vi "pigeon_ver4_1.vi"() -> ()   [LabVIEW 2017]
uses:
  <vilib>/eio/EIONode/EIONode.xnode
  <vilib>/Platform/TimedLoop/XDataNode/XDataNode.xnode
  <vilib>/Platform/TimedLoop/XDataNode/nitl_modes.ctl
  <vilib>/Platform/TimedLoop/XDataNode/XDNodeRunTimeDep.lvlib
  <vilib>/Platform/TimedLoop/XDataNode/wakeup.ctl
  <vilib>/Platform/TimedLoop/XDataNode/timing_clust.ctl
  <vilib>/rvi/DataTransferAndStorage/Container/XNode/niFpgaContainer.xnode
  <vilib>/rvi/eio/common/nirviEmuTemplateMethod_errors.vi
  <vilib>/rvi/Memory/Memory_Emulation/nirvimemoryFastEmulation.vi
  <vilib>/rvi/Memory/Memory_Emulation/nirvimemoryEmulation.vi
  <vilib>/rvi/interface/RandomDataEmulation/nirviRandomDataFpgaReadWriteTemplate.vi
  <vilib>/rvi/Analysis/common/FxpNativeNode/niFpgaFxpNative.xnode
panel:
  out "Numeric":i16
  in  "analog ramp on":bool
  out "AI2":i16
  in  "Tab Control":enum32{"pigeon"}(tab)
  in  "Emergency Stop":bool
  in  "AO0_pigeon":i16
  in  "AO7":i16
  in  "AO6":i16
  out "trigger AI1":bool
  in  "Tab Control 2":T1(tab)
  in  "square wave  on?":bool
  in  "square wave period":i32
  in  "IGBTswitch":bool caption="IGBT Switch circular"
  in  "Manual Override":bool
  in  "circular coil current":i16(slide) scale=0.0..32768.0
  in  "analog ramp period":i16
  in  "AO4":bool
  in  "analog wave shape":i16(ring) items=["Triangle", "Sawtooth", "Sin", ""]
  in  "analog ramp on  2":bool
  in  "End Current":fxp<+,16,16>
  in  "step size":i16=3
  out "ramp loop end?":bool=TRUE
  out "end val 16 bit":i16
  out "ramp start val":fxp<+,15,15>
  out "start val 16 bit":i16
  out "ctr":i16
  out "loop output val":i16
  out "FIFO size":i16
  in  "AO0":i16
  in  "AO1":i16
  in  "AO2":i16
  in  "Run program":bool
  in  "halt processor":bool
  out "control flags":i8 format="%b"
  in  "host operation":i16
  in  "address":u16
  in  "data1":u16
  in  "data2":i32
  in  "repeat program":i32
  out "IP address":i16
  out "PMT1":i16=-4740
  out "ReA":i32
  out "RegB":i16
  out "RegC":i16
  out "exttrigger":bool=TRUE
  out "AI1":i16=161
  out "RegD":i16
  in  "AO4":i16
  in  "AO3":i16
  out "Connector0/AI0":i16
  in  "AO5":i16
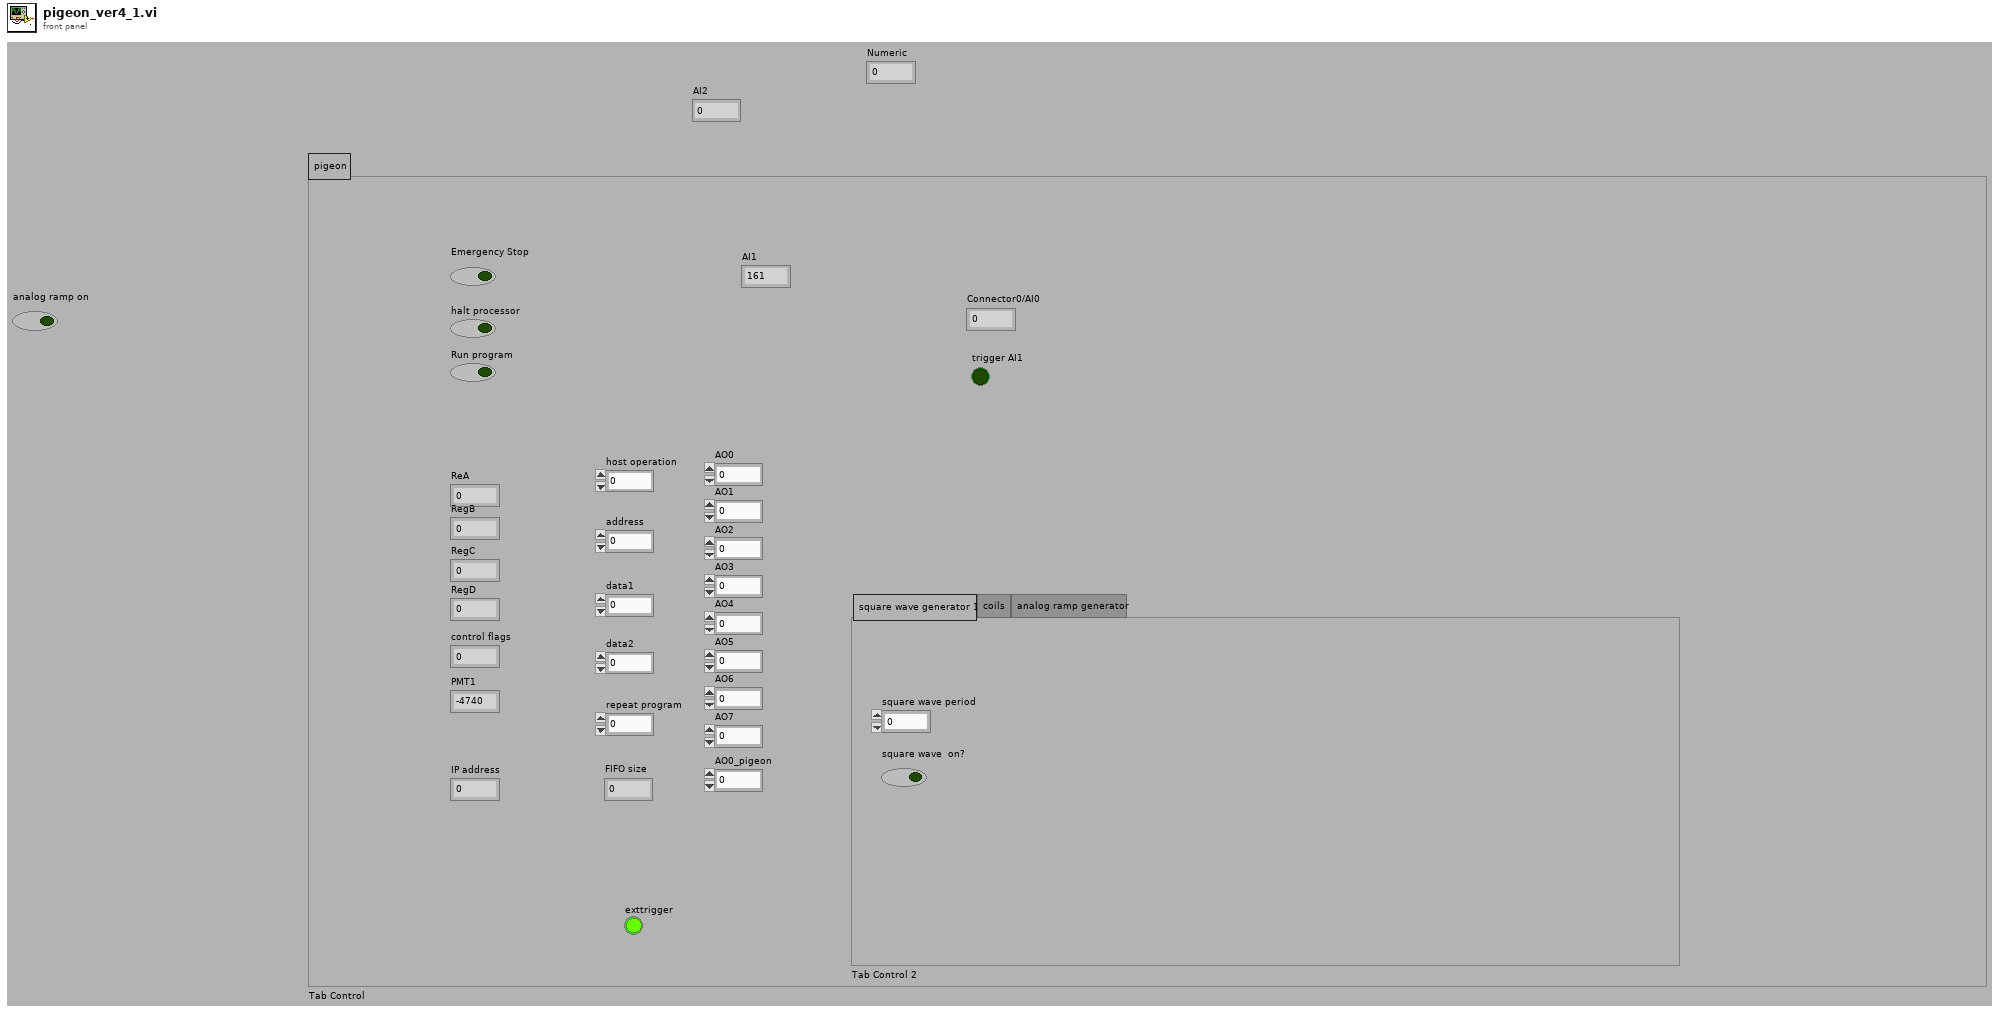
[diagram p1: front panel]
types:
  T1 = enum32{"square wave generator 1", "coils", "analog ramp generator"}
  T2 = typedef "XDNodeRunTimeDep.lvlib/timing_clust.ctl" = cluster{"Expected End [f-1]":u64, "Actual End [f-1]":u64, "Finished Late? [f-1]":bool, "Expected End [i-1]":u64, "Actual End [i-1]":u64, "Finished Late? [i-1]":bool, "Expected Start [i]":u64, "Actual Start [i]":u64, "Expected Start [f]":u64, "Actual Start [f]":u64, "Source Name":string, "Structure Name":string, "Period":i64, "Deadline":i64, "Offset":i64, "Start":i64, "Priority":i32, "Timeout":i32, "Mode":T3, "Wakeup Reason":T4, "Error":errorcluster, "Source Type":string, "Secondary Source Type":string, "Global End Time":u64, "Global Start Time":u64, "Frame Duration":u64, "Iteration Duration":u64, "Assigned CPU":i32, "I/O Scan Engine Mode":u32}
  T3 = typedef "XDNodeRunTimeDep.lvlib/nitl_modes.ctl" = enum32{"No Change", "Process missed periods, maintain original phase", "Discard missed periods, maintain original phase", "Process missed periods, ignore original phase", "Discard missed periods, ignore original phase"}
  T4 = typedef "XDNodeRunTimeDep.lvlib/wakeup.ctl" = enum32{"Normal", "Aborted", "Asynchronous wakeup", "Timing source error", "Timed loop error", "Timeout"}
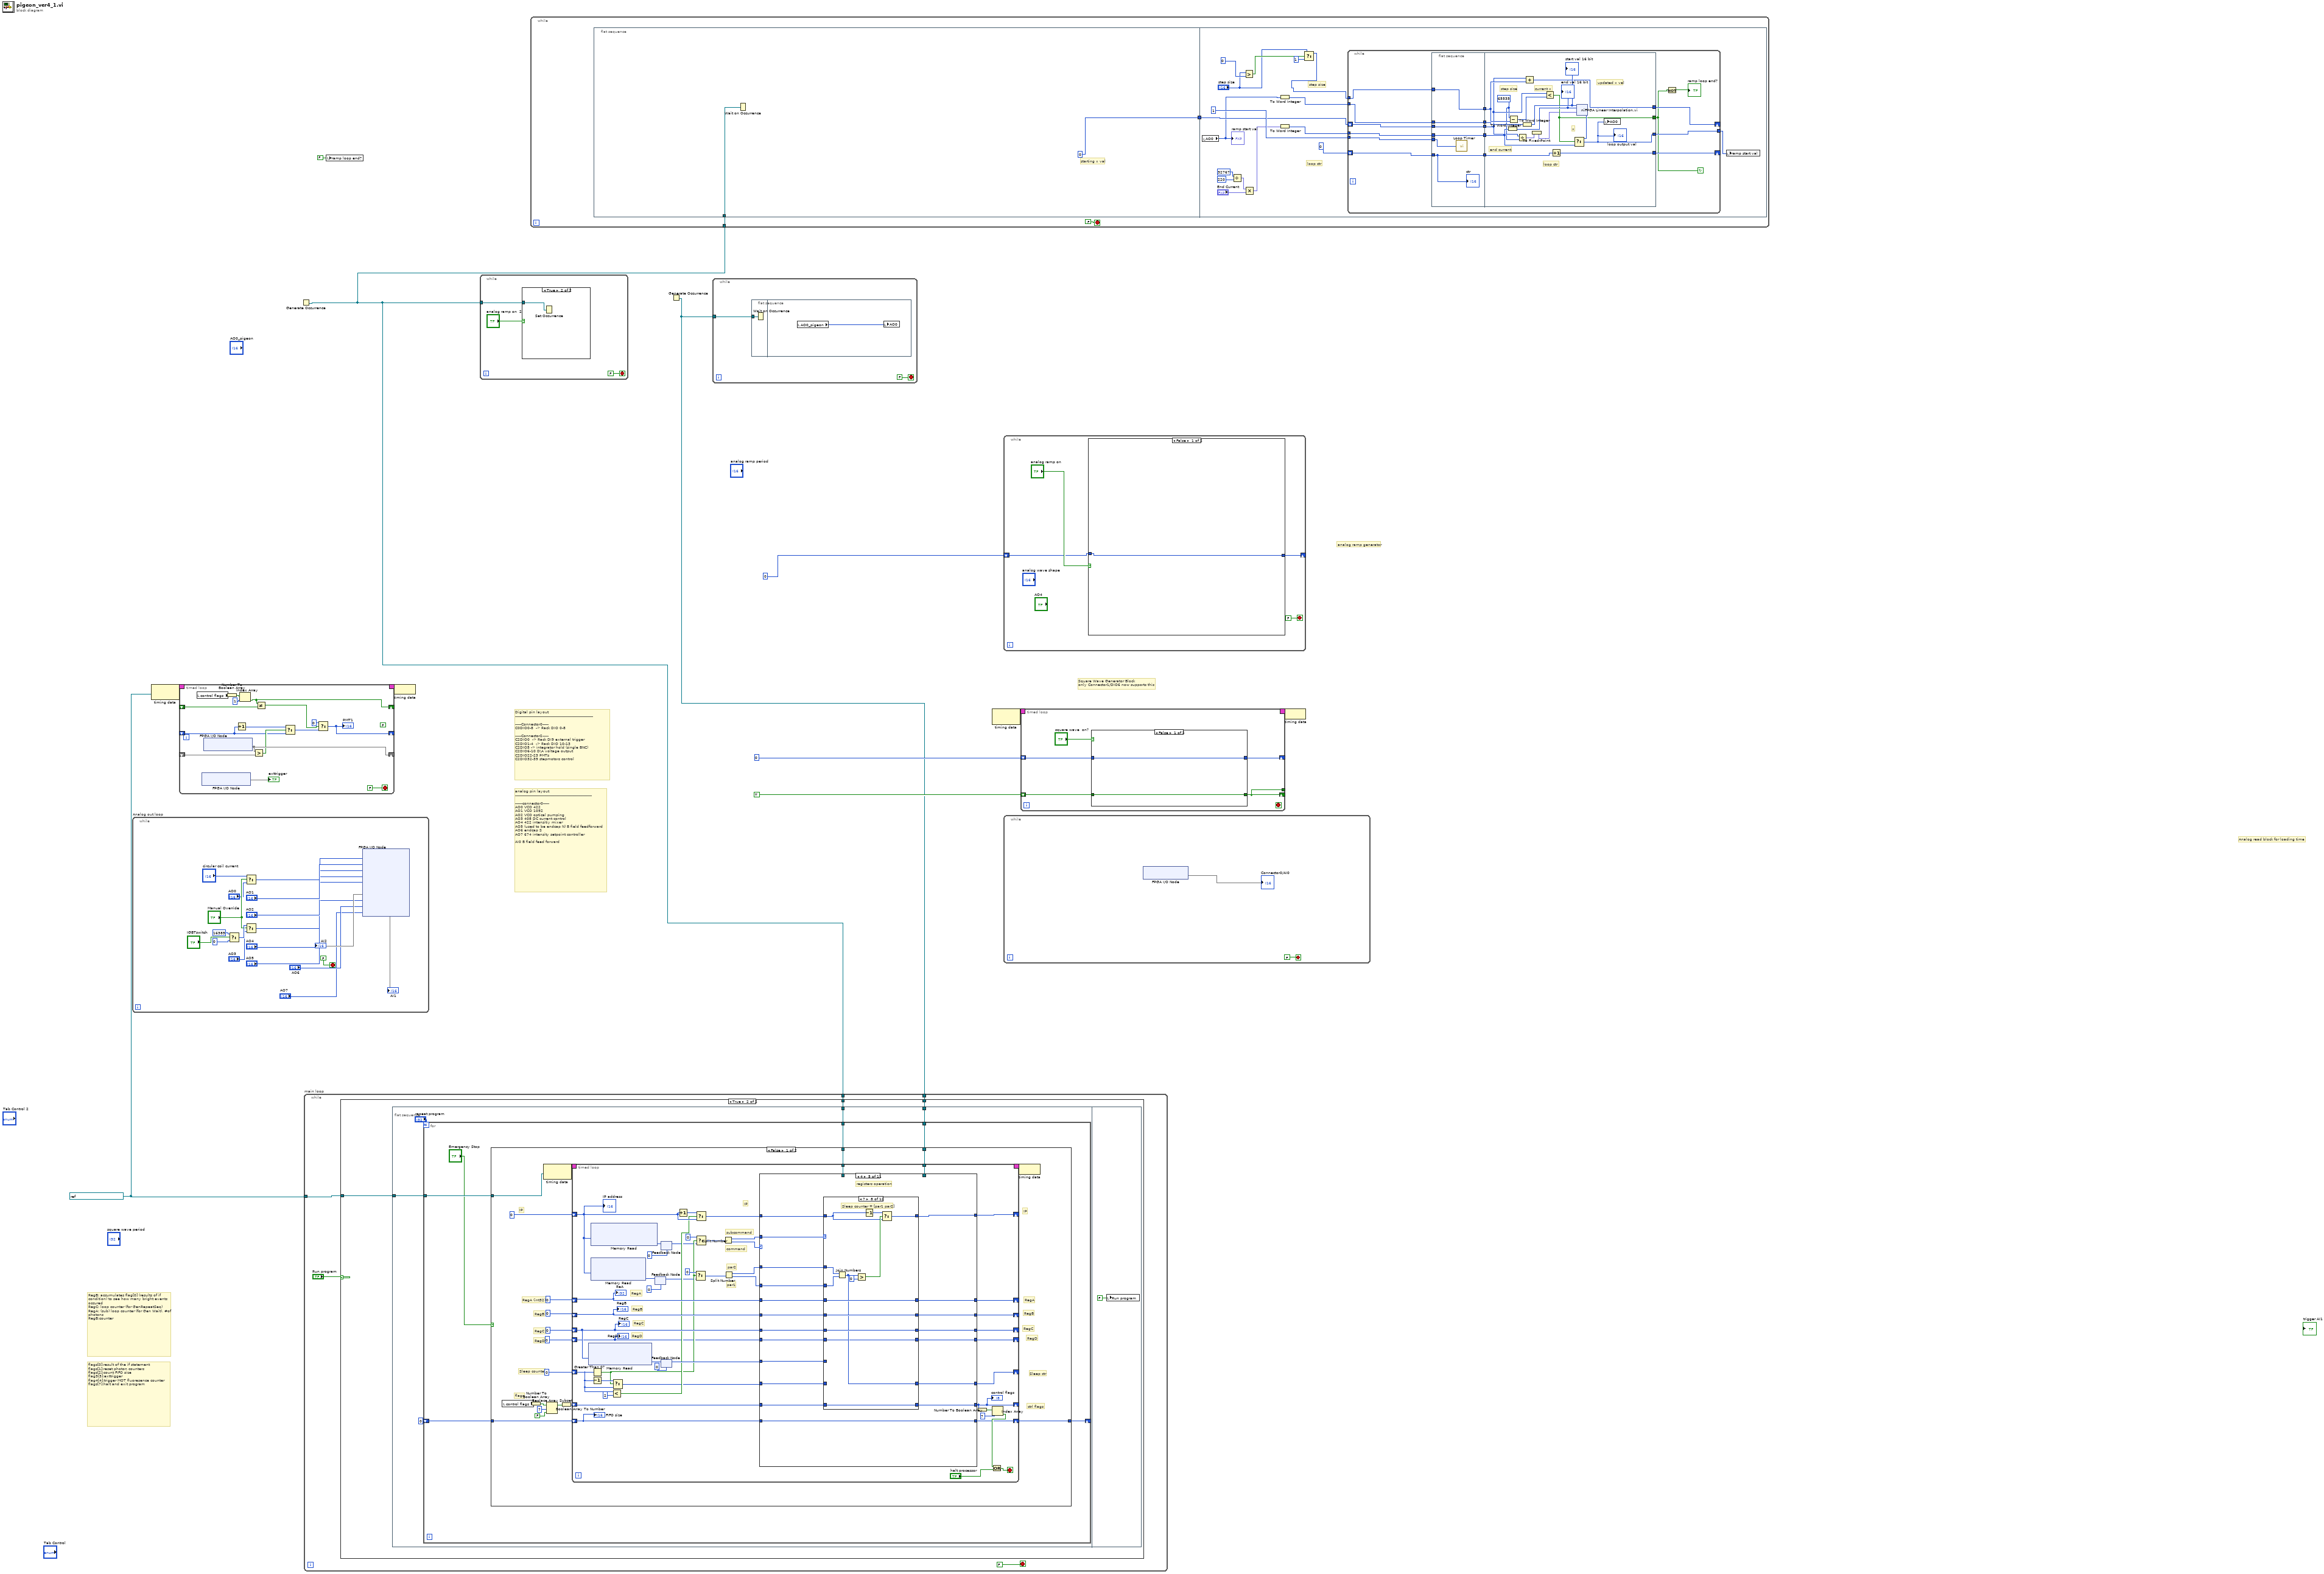
[diagram p0: block diagram]
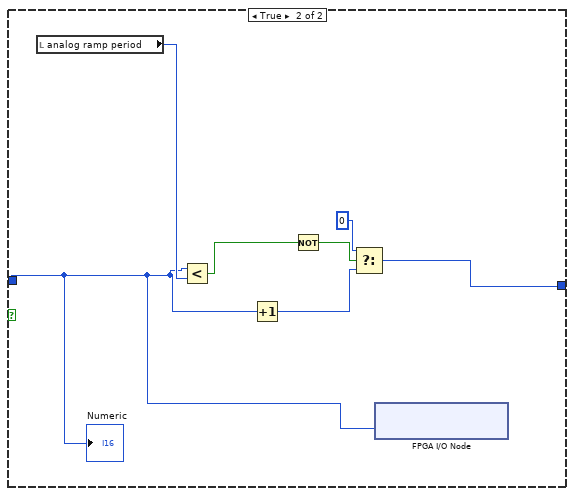
[diagram p3: hidden frame]
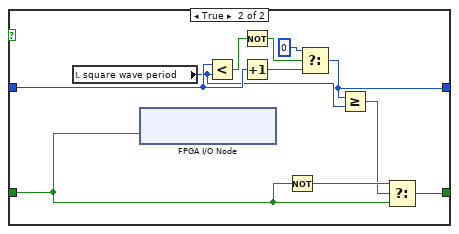
[diagram p4: hidden frame]
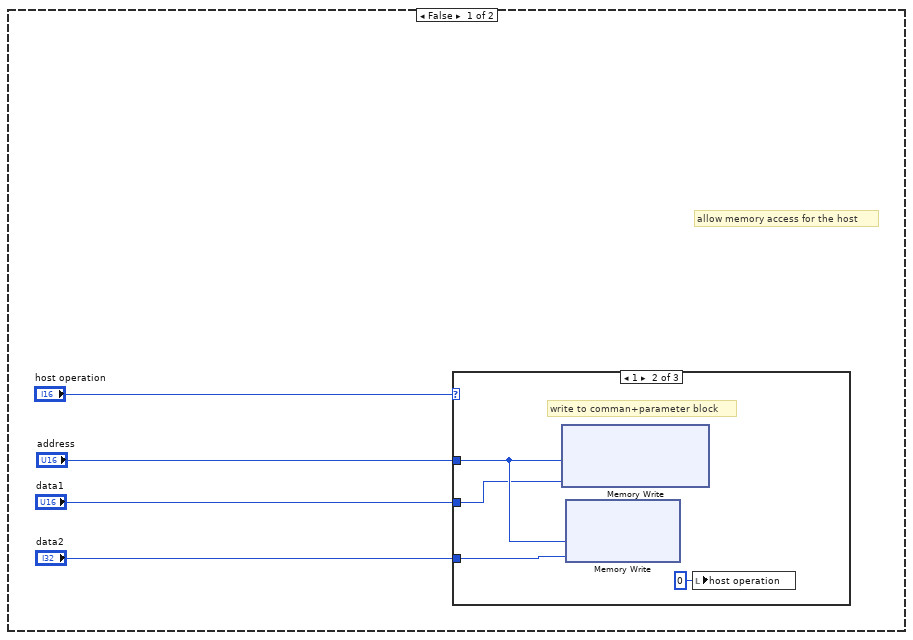
[diagram p5: hidden frame]
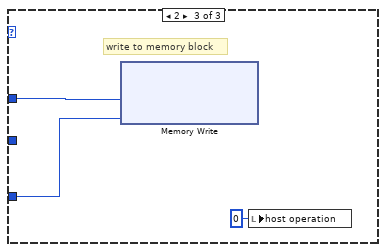
[diagram p7: hidden frame]
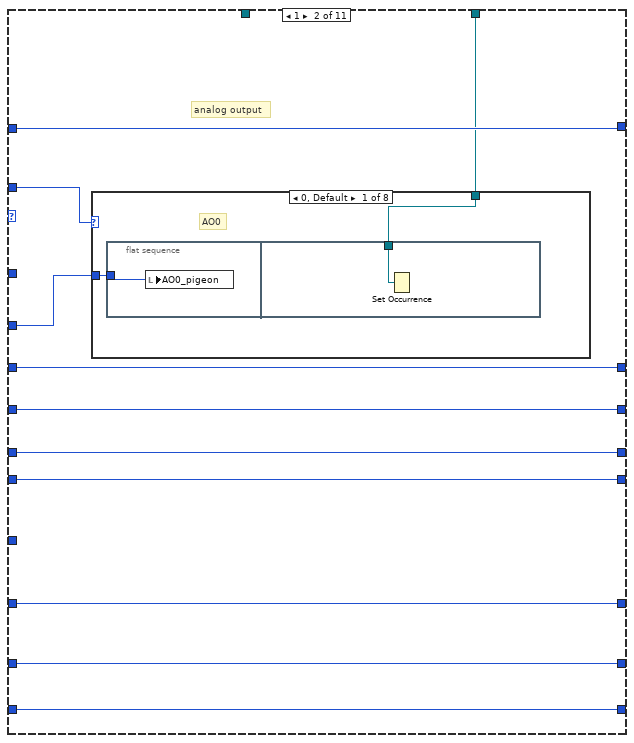
[diagram p9: hidden frame]
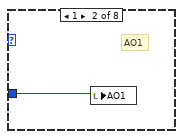
[diagram p10: hidden frame]
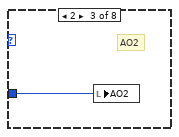
[diagram p11: hidden frame]
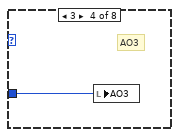
[diagram p12: hidden frame]
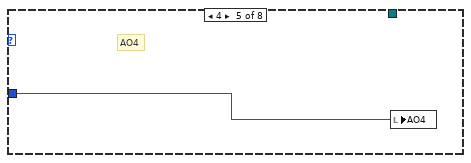
[diagram p13: hidden frame]
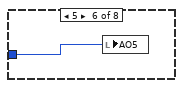
[diagram p14: hidden frame]
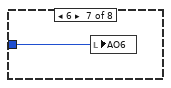
[diagram p15: hidden frame]
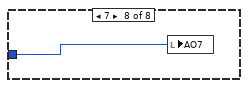
[diagram p16: hidden frame]
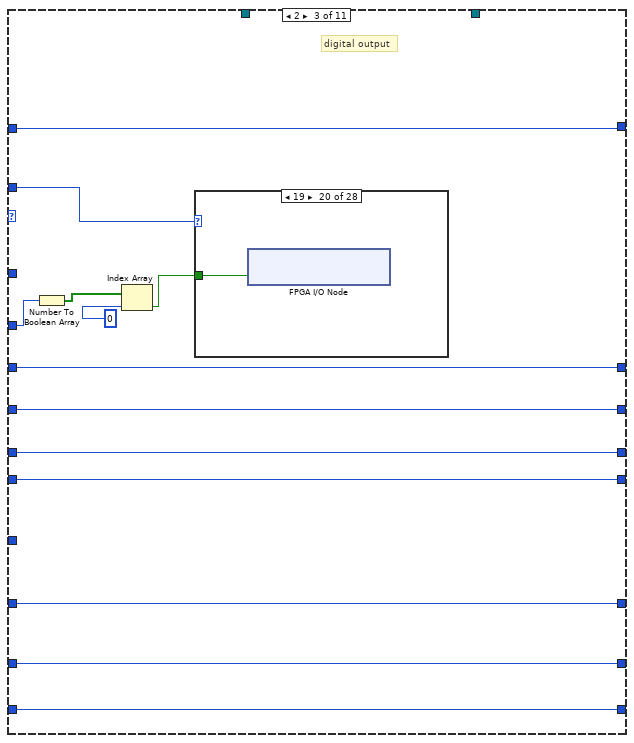
[diagram p17: hidden frame]
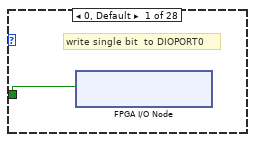
[diagram p18: hidden frame]
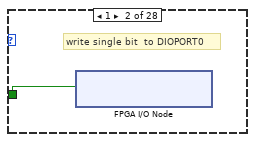
[diagram p19: hidden frame]
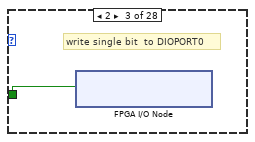
[diagram p20: hidden frame]
diagram:
  w9 = refnum<k21> "40 MHz Onboard Clock" ("FPGA Clock")
  # "analog ramp generator"
  # "Analog read block for loading time"
  # "Square Wave Generator Block\nonly Connector1/DIO6 now supports this"
  # "RegB: accumulates flag[0] (results of if condition) to see how many bright events occured\nRegC: loop counter (for GenRepeatSeq)\nRegA: (sub) loop counter (for Gen Wait), #of     photons \nRegB:counter"
  # "flags[0]:result of the if statement\nflags[1]:reset photon counters\nflags[2]:count FIFO size\nflag3[3]:exttrigger\nflag4[4]:trigger MOT fluoresence counter\nflags[7]:halt and exit program"
  # "Digital pin layout\n----------------------------------------------------------------\n\n-----Connector0-----\nC0DIO0-8  -> Rack DIO 0-8\n\n-----Connector2-----\nC2DIO0  -> Rack DI9 external trigger \nC2DIO1-4  -> Rack DIO 10-13\nC2DIO5 -> integrator hold (single BNC)\nC2DIO6-10 D\\A voltage output\nC2DIO22-23 PMTs\nC2DIO32-39 stepmotors control"
  # "analog pin layout\n---------------------------------------------------------------\n\n------connector0-----\nAO0 VCO 422\nAO1 VCO 1092\nAO2 VCO optical pumping\nAO3 408 DC current control\nAO4 422 intensitiy mixer\nAO5 (used to be endcap N) B field feedforward\nAO6 endcap S\nAO7 674 intensity setpoint controller\n\nAI0 B field feed forward"
  n1 = while "Analog out loop" {
    stop <- FALSE stop-if-true
    n2 = Select(t=i16 16385, s="IGBTswitch", f=i16 0) -> (s? t:f=w20:i16)
    n3 = Select(t="circular coil current", s="Manual Override", f="AO0") -> (s? t:f=w14:i16)
    n4 = Select(t=w20, s="Manual Override", f="AO3") -> (s? t:f=w19:i16)
    n5 = xnode "FPGA I/O Node"("Connector0/AO0"=w14, "Connector0/AO1"="AO1", "Connector0/AO2"="AO2", "Connector0/AO3"=w19, "Connector0/AO4"="AO4", "Connector0/AO5"="AO5", "Connector0/AO6"="AO6", "Connector0/AO7"="AO7") -> ("Connector0/AI1"=→"AI1", "Connector0/AI2"=→"AI2")  [unwired: 10 in, 10 out]
  }
  n6 = node-c288(w9) -> (w11:T2)
  n7 = timed-loop {
    timing: w11 -> [_]
    timing-out: [_] -> w10
    shift-right: [w44] -> _
    shift-left: _ -> [w33]
    shift-right: [w37] -> _
    shift-left: _ -> [w46]
    shift-right: [w39] -> _
    shift-left: _ -> [w40]
    stop <- FALSE stop-if-true
    (unwired) FALSE
    n8 = local read "control flags"() -> (w41:i8)
    n9 = xnode "FPGA I/O Node"() -> ("Connector2/DIO0"=→"exttrigger")  [unwired: 1 in, 1 out]
    n10 = xnode "FPGA I/O Node"() -> ("Connector0/DIO0"=w37)  [unwired: 1 in, 1 out]
    n11 = Number To Boolean Array(number=w41) -> (Boolean array=w42:bool[])
    n12 = Increment(x=w33) -> (x+1=w34:u16)
    n13 = Index Array(array=w42, index=1) -> (element=w39:bool)
    n14 = Greater?(x=w37, y=w46) -> (0:w36:bool)
    n15 = Not Equal?(x=w39, y=w40) -> (x != y?=w31:bool)
    n16 = Select(t=w34, s=w36, f=w33) -> (s? t:f=w45:u16)
    n17 = Select(t=u16 0, s=w31, f=w45) -> (s? t:f=w44:u16)
    "PMT1" <- w44
  }
  n18 = Generate Occurrence() -> (w2:refnum<k4>)
  n19 = local write "ramp loop end?"(FALSE ("ramp loop end?")) -> ()
  n20 = node-c288(w10) -> ()
  n21 = while {
    tunnel: w2 -> [w50]
    stop <- FALSE stop-if-true
    n22 = case shown="True" "analog ramp on  2" {
      tunnel: w50 -> [_ w52]
      frame False {
      }
      frame True {
        n23 = Set Occurrence(w52) -> ()
      }
    }
  }
  n24 = while {
    tunnel: w2 -> [w53]
    stop <- FALSE stop-if-true
    n25 = flat-sequence {
      tunnel: [u16 0] -> w54
      tunnel: w53 -> [w56]
      tunnel: w54 -> [w67]
      frame #0 {
        # "starting x val"
        n26 = Wait on Occurrence(2:w56) -> ()  [unwired: 2 in, 1 out]
      }
      frame #1 {
        # "loop ctr"
        # "step size"
        n27 = local read "AO0"() -> (w58:i16)
        "ramp start val" <- w58
        n28 = Divide(x=i16 32767, y=i16 220) -> (x/y=w72:fxp<+,16,16>)
        n29 = Greater?(x="step size", y=i16 0) -> (0:w62:bool)
        n30 = Multiply(x=w72, y="End Current") -> (x*y=w65:fxp<+,32,32>)
        n31 = To Word Integer(number=w58) -> (16bit integer=w70:i16)
        n32 = To Word Integer(number=w65) -> (16bit integer=w69:i16)
        n33 = Select(t="step size", s=w62, f=i16 1) -> (s? t:f=w59:i16)
        n34 = while {
          tunnel: w59 -> [w78]
          tunnel: w70 -> [w90]
          tunnel: w69 -> [w89]
          shift-right: [w88] -> _
          shift-left: w67 -> [w77]
          tunnel: u32 1 ("Update Period (uSec)") -> [w87]
          shift-right: [w81] -> _
          shift-left: i16 0 -> [w79]
          tunnel: [w80] -> w66
          stop <- w76 continue-if-true
          n35 = flat-sequence {
            tunnel: w78 -> [w95]
            tunnel: [w95] -> w86
            tunnel: w90 -> [w94]
            tunnel: [w94] -> w85
            tunnel: w89 -> [w93]
            tunnel: [w93] -> w84
            tunnel: w77 -> [w92]
            tunnel: [w92] -> w83
            tunnel: w87 -> [w96]
            tunnel: w79 -> [w91]
            tunnel: [w91] -> w82
            tunnel: w86 -> [w104]
            tunnel: w85 -> [w112]
            tunnel: w84 -> [w102]
            tunnel: w83 -> [w100]
            tunnel: [w105] -> w76
            tunnel: [w106] -> w88
            tunnel: [w108] -> w81
            tunnel: w82 -> [w107]
            tunnel: [w97] -> w80
            frame #0 {
              n36 = call "Loop Timer"("Count(uSec)"=w96) -> ()  [unwired: 1 out]
              "ctr" <- w91
            }
            frame #1 {
              w98 = u16 65535 ("x")
              # "current x"
              # "end current"
              # "x"
              # "loop ctr"
              # "updated x val"
              # "step size"
              n37 = To Word Integer(number=w102) -> (16bit integer=w109:i16)
              "end val 16 bit" <- w109
              n38 = Subtract(x=w98, y=w104) -> (x-y=w103:u16)
              n39 = Divide(x=w100, y=w98) -> (x/y=w99:fxp<+,16,0>)
              n40 = To Word Integer(number=w112) -> (16bit integer=w110:i16)
              "start val 16 bit" <- w110
              n41 = Add(x=w100, y=w104) -> (x+y=w106:u16)
              n42 = To Fixed-Point(number=w99) -> (fixed-point=w101:fxp<+,16,0>)  [unwired: 1 in]
              n43 = Less?(x=w100, y=w103) -> (x < y?=w105:bool)
              n44 = Increment(x=w107) -> (x+1=w108:i16)
              n45 = xnode ("niFPGA Linear Interpolation.vi")("y0"=w110, "y1"=w109, "x"=w101) -> ("y"=w111:i16)
              n46 = Select(t=w111, s=w105, f=w102) -> (s? t:f=w97:i16)
              "loop output val" <- w97
              n47 = local write "AO0"(w97) -> ()
            }
          }
          n48 = Not(x=w76) -> (.not. x?=→"ramp loop end?":bool)
        }
        n49 = local write "ramp start val"(w66) -> ()
      }
    }
  }
  n50 = Generate Occurrence() -> (w1:refnum<k4>)
  n51 = while "main loop" {
    tunnel: w9 -> [w126]
    tunnel: w2 -> [w125]
    tunnel: w1 -> [w124]
    stop <- FALSE ("stop") stop-if-true
    n52 = case shown="True" "Run program" {
      tunnel: w126 -> [_ w142]
      tunnel: w125 -> [_ w141]
      tunnel: w124 -> [_ w140]
      frame False {
        # "allow memory access for the host"
        n53 = case shown="1" "host operation" {
          tunnel: "address" -> [_ w134 w139]
          tunnel: "data1" -> [_ w133 _]
          tunnel: "data2" -> [_ w136 w137]
          frame 0, Default {
          }
          frame 1 {
            # "write to comman+parameter block"
            n54 = xnode ("Memory Write")("Address"=w134, "Data"=w133) -> ()  [unwired: 1 in, 1 out]
            n55 = xnode ("Memory Write")("Address"=w134, "Data"=w136) -> ()  [unwired: 1 in, 1 out]
            n56 = local write "host operation"(i16 0 ("host operation")) -> ()
          }
          frame 2 {
            # "write to memory block"
            n57 = xnode ("Memory Write")("Address"=w139, "Data"=w137) -> ()  [unwired: 1 in, 1 out]
            n58 = local write "host operation"(i16 0 ("host operation")) -> ()
          }
        }
      }
      frame True {
        n59 = flat-sequence {
          tunnel: w142 -> [w146]
          tunnel: w141 -> [w144]
          tunnel: w140 -> [w143]
          frame #0 {
            n60 = for {
              N: "repeat program" -> [_]
              tunnel: w146 -> [w153]
              shift-right: [w151] -> _
              shift-left: i16 0 -> [w152]
              tunnel: w144 -> [w150]
              tunnel: w143 -> [w149]
              n61 = case shown="False" "Emergency Stop" {
                tunnel: w153 -> [w166 _]
                tunnel: w152 -> [w158 w630]
                tunnel: [w157 w630] -> w151
                tunnel: w150 -> [w155 _]
                tunnel: w149 -> [w154 _]
                frame False {
                  # "ctrl flags"
                  # "Sleep ctr"
                  # "RegD"
                  # "RegD"
                  # "Sleep counter"
                  # "flags"
                  # "RegC"
                  # "RegB"
                  # "RegA"
                  # "RegC"
                  # "RegB"
                  # "RegA (int32)"
                  # "IP"
                  # "IP"
                  n62 = local read "control flags"() -> (w161:i8)
                  n63 = Number To Boolean Array(number=w161) -> (Boolean array=w165:bool[])
                  n64 = node-c288(w166) -> (w172:T2)
                  n65 = Replace Array Subset(array=w165, new element=FALSE ("new element/subarray"), index=7) -> (w163:bool[])
                  n66 = Boolean Array To Number(Boolean array=w163) -> (number=w164:u8)
                  n67 = timed-loop {
                    timing: w172 -> [_]
                    timing-out: [_] -> w171
                    shift-right: [w209] -> _
                    shift-left: i16 0 -> [w192]
                    shift-right: [w205] -> _
                    shift-left: 0 -> [w201]
                    shift-right: [w217] -> _
                    shift-left: i16 0 -> [w208]
                    shift-right: [w216] -> _
                    shift-left: i16 0 -> [w200]
                    shift-right: [w206] -> _
                    shift-left: w164 -> [w207]
                    shift-right: [w199] -> _
                    shift-left: i16 0 -> [w190]
                    shift-right: [w181] -> w157
                    shift-left: w158 -> [w180]
                    shift-right: [w178] -> _
                    shift-left: i16 0 -> [w179]
                    tunnel: w155 -> [w174]
                    tunnel: w154 -> [w173]
                    stop <- w212 stop-if-true
                    # "RegD"
                    # "IP"
                    # "RegC"
                    # "RegB"
                    # "RegA"
                    # "par1"
                    # "par2"
                    # "subcommand"
                    # "command"
                    n68 = xnode ("Memory Read")("Address"=w200) -> ("Data"=w204:i16)  [unwired: 2 in, 2 out]
                    n69 = xnode ("Memory Read")("Address"=w192) -> ("Data"=w187:u16)  [unwired: 1 in, 1 out]
                    n70 = xnode ("Memory Read")("Address"=w192) -> ("Data"=w183:i32)  [unwired: 1 in, 1 out]
                    n71 = Greater Than 0?(x=w190) -> (x > 0?=w185:bool)
                    n72 = Decrement(x=w190) -> (x-1=w191:u32)
                    n73 = Less?(x=w190, y=u32 2) -> (x < y?=w189:bool)
                    n74 = Select(t=w191, s=w185, f=w190) -> (s? t:f=w188:u32)
                    n75 = feedback-in #1(w183) -> ()
                    n76 = feedback #1(u32 0 ("Data")) -> (w182:u32)
                    n77 = feedback-in #2(w204) -> ()
                    n78 = feedback #2(0) -> (w203:i32)
                    n79 = feedback-in #3(w187) -> ()
                    n80 = feedback #3(u16 0 ("Data")) -> (w184:u16)
                    n81 = Increment(x=w192) -> (x+1=w193:u16)
                    n82 = Select(t=0, s=w185, f=w182) -> (s? t:f=w196:u32)
                    n83 = Select(t=w193, s=w189, f=w192) -> (s? t:f=w198:u16)
                    n84 = Select(t=u16 0, s=w185, f=w184) -> (s? t:f=w197:u16)
                    n85 = Split Number(x=w197) -> (hi(x)=w218:u8, lo(x)=w219:u8)
                    n86 = Split Number(x=w196) -> (hi(x)=w210:u16, lo(x)=w211:u16)
                    n87 = case shown="4" w219 {
                      tunnel: w211 -> [_ w237 w254 _ w334 w454 w528 _ _ w588 _]
                      tunnel: w210 -> [_ _ _ _ w327 w453 w527 _ _ w589 _]
                      tunnel: w218 -> [_ w238 w262 w301 w335 w458 _ w546 _ w570 _]
                      tunnel: w201 -> [w227 w236 w261 w293 w333 w455 w532 w550 w566 w587 w617]
                      tunnel: [w227 w236 w261 w293 w330 w455 w532 w550 w566 w586 w617] -> w205
                      tunnel: w208 -> [w226 w235 w260 w292 w332 w456 w533 w549 w569 w585 w618]
                      tunnel: w200 -> [w225 w234 w259 w299 w331 w457 w534 w548 w568 w583 w619]
                      tunnel: [w226 w235 w260 w291 w329 w456 w533 w549 w569 w584 w618] -> w217
                      tunnel: [w225 w234 w259 w299 w328 w457 w534 w548 w568 w582 w619] -> w216
                      tunnel: [w223 w233 w258 w300 w323 w461 w526 w552 w567 w572 w616] -> w209
                      tunnel: w198 -> [w223 w233 w258 w300 w324 w461 _ w552 w567 w573 w616]
                      tunnel: [w224 w232 w257 w297 w325 w460 w525 w541 w563 w576 w622] -> w206
                      tunnel: w207 -> [w224 w232 w257 w298 w326 w459 w525 w540 w562 w577 w622]
                      tunnel: w203 -> [_ _ _ _ w317 w452 _ _ _ _ _]
                      tunnel: w188 -> [w222 w231 w252 w296 w322 w451 w524 w538 w559 w579 w623]
                      tunnel: [w222 w231 w252 w296 w321 w451 w524 w538 w559 w578 w623] -> w199
                      tunnel: w180 -> [w221 w230 w251 w295 w320 w450 w523 w537 w558 w574 w621]
                      tunnel: [w221 w230 w251 w295 w320 w450 w523 w536 w558 w575 w621] -> w181
                      tunnel: w179 -> [w220 w229 w250 w294 w319 w449 w522 w535 w557 w581 w620]
                      tunnel: [w220 w229 w250 w294 w318 w449 w522 w535 w557 w580 w620] -> w178
                      tunnel: w174 -> [_ _ _ _ _ _ _ _ _ w571 _]
                      tunnel: w173 -> [_ w228 _ _ _ _ _ _ _ _ _]
                      frame 0, Default {
                      }
                      frame 1 {
                        # "analog output"
                        n88 = case shown="0, Default" w238 {
                          tunnel: w237 -> [w240 w243 w244 w245 w246 w247 w248 w249]
                          tunnel: w228 -> [w239 _ _ _ _ _ _ _]
                          frame 0, Default {
                            # "AO0"
                            n89 = flat-sequence {
                              tunnel: w240 -> [w241]
                              tunnel: w239 -> [w242]
                              frame #0 {
                                n90 = local write "AO0_pigeon"(w241) -> ()
                              }
                              frame #1 {
                                n91 = Set Occurrence(w242) -> ()
                              }
                            }
                          }
                          frame 1 {
                            # "AO1"
                            n92 = local write "AO1"(w243) -> ()
                          }
                          frame 2 {
                            # "AO2"
                            n93 = local write "AO2"(w244) -> ()
                          }
                          frame 3 {
                            # "AO3"
                            n94 = local write "AO3"(w245) -> ()
                          }
                          frame 4 {
                            # "AO4"
                            n95 = local write "AO4"(w246) -> ()
                          }
                          frame 5 {
                            n96 = local write "AO5"(w247) -> ()
                          }
                          frame 6 {
                            n97 = local write "AO6"(w248) -> ()
                          }
                          frame 7 {
                            n98 = local write "AO7"(w249) -> ()
                          }
                        }
                      }
                      frame 2 {
                        # "digital output"
                        n99 = Number To Boolean Array(number=w254) -> (Boolean array=w255:bool[])
                        n100 = Index Array(array=w255, index=0) -> (element=w253:bool)
                        n101 = case shown="19" w262 {
                          tunnel: w253 -> [w263 w264 w265 w266 w267 w268 w269 w270 w271 w272 w273 w274 w275 w276 w277 w278 w279 w280 w281 w282 w283 w284 w285 w286 w287 w288 w289 w290]
                          frame 0, Default {
                            # "write single bit  to DIOPORT0"
                            n102 = xnode "FPGA I/O Node"("Connector1/DIO0"=w263) -> ()  [unwired: 1 in, 1 out]
                          }
                          frame 1 {
                            # "write single bit  to DIOPORT0"
                            n103 = xnode "FPGA I/O Node"("Connector1/DIO1"=w264) -> ()  [unwired: 1 in, 1 out]
                          }
                          frame 2 {
                            # "write single bit  to DIOPORT0"
                            n104 = xnode "FPGA I/O Node"("Connector1/DIO2"=w265) -> ()  [unwired: 1 in, 1 out]
                          }
                          frame 3 {
                            # "write single bit  to DIOPORT0"
                            n105 = xnode "FPGA I/O Node"("Connector1/DIO3"=w266) -> ()  [unwired: 1 in, 1 out]
                          }
                          frame 4 {
                            # "write single bit  to DIOPORT0"
                            n106 = xnode "FPGA I/O Node"("Connector1/DIO4"=w267) -> ()  [unwired: 1 in, 1 out]
                          }
                          frame 5 {
                            # "write single bit  to DIOPORT0"
                            n107 = xnode "FPGA I/O Node"("Connector1/DIO5"=w268) -> ()  [unwired: 1 in, 1 out]
                          }
                          frame 6 {
                            # "write single bit  to DIOPORT0"
                            n108 = xnode "FPGA I/O Node"("Connector1/DIO6"=w269) -> ()  [unwired: 1 in, 1 out]
                          }
                          frame 7 {
                            # "write single bit  to DIOPORT0"
                            n109 = xnode "FPGA I/O Node"("Connector1/DIO7"=w270) -> ()  [unwired: 1 in, 1 out]
                          }
                          frame 8 {
                            # "write single bit  to DIOPORT0"
                            n110 = xnode "FPGA I/O Node"("Connector1/DIO8"=w271) -> ()  [unwired: 1 in, 1 out]
                          }
                          frame 9 {
                            n111 = xnode "FPGA I/O Node"("Connector1/DIO9"=w272) -> ()  [unwired: 1 in, 1 out]
                          }
                          frame 10 {
                            n112 = xnode "FPGA I/O Node"("Connector1/DIO10"=w273) -> ()  [unwired: 1 in, 1 out]
                          }
                          frame 11 {
                            n113 = xnode "FPGA I/O Node"("Connector1/DIO11"=w274) -> ()  [unwired: 1 in, 1 out]
                          }
                          frame 12 {
                            n114 = xnode "FPGA I/O Node"("Connector1/DIO12"=w275) -> ()  [unwired: 1 in, 1 out]
                          }
                          frame 13 {
                            n115 = xnode "FPGA I/O Node"("Connector1/DIO13"=w276) -> ()  [unwired: 1 in, 1 out]
                          }
                          frame 14 {
                            n116 = xnode "FPGA I/O Node"("Connector1/DIO14"=w277) -> ()  [unwired: 1 in, 1 out]
                          }
                          frame 15 {
                            n117 = xnode "FPGA I/O Node"("Connector1/DIO15"=w278) -> ()  [unwired: 1 in, 1 out]
                          }
                          frame 16 {
                            n118 = xnode "FPGA I/O Node"("Connector1/DIO16"=w279) -> ()  [unwired: 1 in, 1 out]
                          }
                          frame 17 {
                            n119 = xnode "FPGA I/O Node"("Connector1/DIO17"=w280) -> ()  [unwired: 1 in, 1 out]
                          }
                          frame 18 {
                            n120 = xnode "FPGA I/O Node"("Connector1/DIO18"=w281) -> ()  [unwired: 1 in, 1 out]
                          }
                          frame 19 {
                            n121 = xnode "FPGA I/O Node"("Connector1/DIO19"=w282) -> ()  [unwired: 1 in, 1 out]
                          }
                          frame 20 {
                            n122 = xnode "FPGA I/O Node"("Connector2/DIO12"=w283) -> ()  [unwired: 1 in, 1 out]
                          }
                          frame 21 {
                            n123 = xnode "FPGA I/O Node"("Connector2/DIO17"=w284) -> ()  [unwired: 1 in, 1 out]
                          }
                          frame 22 {
                            n124 = xnode "FPGA I/O Node"("Connector2/DIO19"=w285) -> ()  [unwired: 1 in, 1 out]
                          }
                          frame 23 {
                            n125 = xnode "FPGA I/O Node"("Connector2/DIO18"=w286) -> ()  [unwired: 1 in, 1 out]
                          }
                          frame 24 {
                            n126 = xnode "FPGA I/O Node"("Connector2/DIO21"=w287) -> ()  [unwired: 1 in, 1 out]
                          }
                          frame 25 {
                            n127 = xnode "FPGA I/O Node"("Connector2/DIO24"=w288) -> ()  [unwired: 1 in, 1 out]
                          }
                          frame 26 {
                            n128 = xnode "FPGA I/O Node"("Connector2/DIO25"=w289) -> ()  [unwired: 1 in, 1 out]
                          }
                          frame 27 {
                            n129 = xnode "FPGA I/O Node"("Connector2/DIO20"=w290) -> ()  [unwired: 1 in, 1 out]
                          }
                        }
                      }
                      frame 3 {
                        # "photon counting"
                        n130 = case shown="3" w301 {
                          tunnel: [w302 w304 w316] -> w291
                          tunnel: w292 -> [w302 w305 w316]
                          tunnel: w298 -> [w303 w307 w314]
                          tunnel: [w303 w307 w313] -> w297
                          frame 2, Default {
                          }
                          frame 1 {
                            # "PMT1"
                            n131 = local read "PMT1"() -> (w306:i16)
                            n132 = Add(x=w306, y=w305) -> (x+y=w304:u16)
                          }
                          frame 3 {
                            # "Reset  photon counter"
                            # "make a Not gate of flag(1)"
                            n133 = Number To Boolean Array(number=w314) -> (Boolean array=w311:bool[])
                            n134 = Index Array(array=w311, index=1) -> (element=w309:bool)
                            n135 = Not(x=w309) -> (.not. x?=w308:bool)
                            n136 = Replace Array Subset(array=w311, new element=w308, index=1) -> (w312:bool[])
                            n137 = Boolean Array To Number(Boolean array=w312) -> (number=w313:u8)
                          }
                        }
                      }
                      frame 4 {
                        # "registers operation"
                        n138 = case shown="7" w335 {
                          tunnel: w334 -> [w341 w351 w358 _ _ _ _ w400 _ _ w427 w440]
                          tunnel: w333 -> [_ w350 w357 w364 w372 w380 w384 w405 w416 w422 w432 w445]
                          tunnel: w332 -> [w344 _ w356 w363 w374 w379 w392 w404 w415 w418 w430 w443]
                          tunnel: w331 -> [w343 w349 _ w366 w373 _ w385 w403 w414 w421 w431 w444]
                          tunnel: [w340 w350 w357 w364 w371 w380 w384 w405 w416 w422 w432 w445] -> w330
                          tunnel: [w344 w351 w356 w363 w374 w379 w391 w404 w415 w420 w430 w443] -> w329
                          tunnel: [w343 w349 w358 w365 w373 w379 w385 w403 w414 w421 w431 w444] -> w328
                          tunnel: w327 -> [w342 _ _ _ _ _ _ w401 _ _ _ w439]
                          tunnel: w326 -> [w339 w348 w355 w362 w370 w378 w386 w402 w413 w425 w435 w448]
                          tunnel: [w339 w348 w355 w362 w370 w378 w386 w402 w413 w425 w435 w448] -> w325
                          tunnel: w324 -> [w338 w347 w354 w361 w369 w377 w383 w394 w408 w424 w434 w447]
                          tunnel: [w338 w347 w354 w361 w369 w377 w383 w397 w411 w424 w434 w447] -> w323
                          tunnel: w322 -> [w337 w346 w353 w360 w368 w376 w382 _ _ w423 w433 w446]
                          tunnel: [w337 w346 w353 w360 w368 w376 w382 w398 w406 w423 w433 w446] -> w321
                          tunnel: w319 -> [w336 w345 w352 w359 w367 w375 w381 w393 w407 w417 _ w438]
                          tunnel: [w336 w345 w352 w359 w367 w375 w381 w393 w407 w417 w428 w437] -> w318
                          tunnel: w317 -> [_ _ _ _ _ _ _ _ w406 _ _ _]
                          frame 0, Default {
                            # "Set par1,2 to RegA"
                            n139 = Join Numbers(hi=w342, lo=w341) -> ((hi.lo)=w340:u32)
                          }
                          frame 1 {
                            # "Set par1 to RegB"
                          }
                          frame 2 {
                            # "Set par1 to RegC"
                          }
                          frame 3 {
                            # "increase RegC by 1"
                            n140 = Increment(x=w366) -> (x+1=w365:u16)
                          }
                          frame 4 {
                            # "increase RegA by 1"
                            n141 = Increment(x=w372) -> (x+1=w371:u32)
                          }
                          frame 5 {
                            # "Set regC to regB"
                          }
                          frame 6 {
                            # "regB<-regB+flags[0]"
                            n142 = Number To Boolean Array(number=w386) -> (Boolean array=w390:bool[])
                            n143 = Index Array(array=w390, index=0) -> (element=w388:bool)
                            n144 = Boolean To (0,1)(Boolean=w388) -> (0, 1=w387:i16)
                            n145 = Add(x=w387, y=w392) -> (x+y=w391:u16)
                          }
                          frame 7 {
                            # "Sleep counter = [par1 par2]"
                            n146 = Join Numbers(hi=w401, lo=w400) -> ((hi.lo)=w398:u32)
                            n147 = Greater?(x=w398, y=u32 0) -> (0:w396:bool)
                            n148 = Decrement(x=w394) -> (x-1=w395:u16)
                            n149 = Select(t=w395, s=w396, f=w394) -> (s? t:f=w397:u16)
                          }
                          frame 11 {
                            # "Sleep counter =par1* memory Block[RegC]"
                            n150 = Greater?(x=w406, y=u32 0) -> (0:w410:bool)
                            n151 = Decrement(x=w408) -> (x-1=w409:u16)
                            n152 = Select(t=w409, s=w410, f=w408) -> (s? t:f=w411:u16)
                          }
                          frame 8 {
                            # "RegB=RegB+ RegA(lo)"
                            n153 = Split Number(x=w422) -> (lo(x)=w419:u16)  [unwired: 1 out]
                            n154 = Add(x=w419, y=w418) -> (x+y=w420:u16)
                          }
                          frame 9 {
                            # "RegD<-AI1+par1"
                            n155 = To Word Integer(number=w427) -> (16bit integer=w426:i16)
                            n156 = local read "AI1"() -> (w429:i16)
                            n157 = Add(x=w426, y=w429) -> (x+y=w428:i16)
                          }
                          frame 10 {
                            # "RegD<-RegD*2^par1*par2"
                            n158 = To Word Integer(number=w439) -> (16bit integer=w441:i16)
                            n159 = To Word Integer(number=w440) -> (16bit integer=w442:i16)
                            n160 = Multiply(x=w441, y=w438) -> (x*y=w436:i16)
                            n161 = Scale By Power Of 2(n=w442, x=w436) -> (x*2^n=w437:i16)
                          }
                        }
                      }
                      frame 5 {
                        # "If statement"
                        n162 = case shown="4" w458 {
                          tunnel: [w471 w479 w487 w495 w505 w508 w516] -> w460
                          tunnel: w459 -> [w470 w478 w486 w494 w504 w509 w517]
                          tunnel: w453 -> [w464 _ _ _ _ _ _]
                          tunnel: w457 -> [_ _ w482 w489 _ _ _]
                          tunnel: w456 -> [_ w473 _ w488 _ _ _]
                          tunnel: w455 -> [w465 _ _ _ _ w506 w514]
                          tunnel: w454 -> [w463 w472 w481 _ _ w507 _]
                          tunnel: w452 -> [_ _ _ _ _ _ w521]
                          frame 0, Default {
                            # "The if regA =  [par1,par2]"
                            n163 = Number To Boolean Array(number=w470) -> (Boolean array=w468:bool[])
                            n164 = Join Numbers(hi=w464, lo=w463) -> ((hi.lo)=w462:u32)
                            n165 = Equal?(x=w462, y=w465) -> (x = y?=w466:bool)
                            n166 = Replace Array Subset(array=w468, new element=w466, index=0) -> (w467:bool[])
                            n167 = Boolean Array To Number(Boolean array=w467) -> (number=w471:u8)
                          }
                          frame 1 {
                            # "The if  regB >  par1"
                            n168 = Number To Boolean Array(number=w478) -> (Boolean array=w476:bool[])
                            n169 = Greater?(x=w473, y=w472) -> (0:w474:bool)
                            n170 = Replace Array Subset(array=w476, new element=w474, index=0) -> (w475:bool[])
                            n171 = Boolean Array To Number(Boolean array=w475) -> (number=w479:u8)
                          }
                          frame 2 {
                            # "The if  regC=  par1"
                            n172 = Number To Boolean Array(number=w486) -> (Boolean array=w484:bool[])
                            n173 = Equal?(x=w481, y=w482) -> (x = y?=w480:bool)
                            n174 = Replace Array Subset(array=w484, new element=w480, index=0) -> (w483:bool[])
                            n175 = Boolean Array To Number(Boolean array=w483) -> (number=w487:u8)
                          }
                          frame 3 {
                            # "The if  regB> regC"
                            n176 = Number To Boolean Array(number=w494) -> (Boolean array=w492:bool[])
                            n177 = Greater?(x=w488, y=w489) -> (0:w490:bool)
                            n178 = Replace Array Subset(array=w492, new element=w490, index=0) -> (w491:bool[])
                            n179 = Boolean Array To Number(Boolean array=w491) -> (number=w495:u8)
                          }
                          frame 4 {
                            w500 = 3 ("index")
                            # "external trigger rising edge"
                            n180 = Number To Boolean Array(number=w504) -> (Boolean array=w501:bool[])
                            n181 = local read "exttrigger"() -> (w497:bool)
                            n182 = Index Array(array=w501, index=w500) -> (element=w499:bool)
                            n183 = Not(x=w499) -> (.not. x?=w498:bool)
                            n184 = And(x=w497, y=w498) -> (x .and. y?=w496:bool)
                            n185 = Replace Array Subset(array=w501, new element #1=w496, index #1=0 ("index"), new element #2=w497, index #2=w500) -> (w502:bool[])
                            n186 = Boolean Array To Number(Boolean array=w502) -> (number=w505:u8)
                          }
                          frame 5 {
                            # "The if  regA >  par1"
                            n187 = Number To Boolean Array(number=w509) -> (Boolean array=w512:bool[])
                            n188 = Greater?(x=w506, y=w507) -> (0:w510:bool)
                            n189 = Replace Array Subset(array=w512, new element=w510, index=0) -> (w511:bool[])
                            n190 = Boolean Array To Number(Boolean array=w511) -> (number=w508:u8)
                          }
                          frame 6 {
                            # "The if  regA == memoryBlock(regC)"
                            n191 = Number To Boolean Array(number=w517) -> (Boolean array=w519:bool[])
                            n192 = Equal?(x=w514, y=w521) -> (x = y?=w515:bool)
                            n193 = Replace Array Subset(array=w519, new element=w515, index=0) -> (w518:bool[])
                            n194 = Boolean Array To Number(Boolean array=w518) -> (number=w516:u8)
                          }
                        }
                      }
                      frame 6 {
                        # "condition (flags[0]) goto\nuse par1=par2 for normal goto"
                        n195 = Number To Boolean Array(number=w525) -> (Boolean array=w531:bool[])
                        n196 = Index Array(array=w531, index=0) -> (element=w529:bool)
                        n197 = Select(t=w528, s=w529, f=w527) -> (s? t:f=w526:u16)
                      }
                      frame 7 {
                        w539 = 2 ("index")
                        # "make a Not gate of flag(2)"
                        # "push  to FIFO"
                        n198 = case shown="4" w546 {
                          tunnel: w550 -> [w553 _ _ _]
                          tunnel: w549 -> [_ w554 _ _]
                          tunnel: w548 -> [_ _ w555 _]
                          tunnel: [w553 w554 w555 w556] -> w547
                          frame 0, Default {
                            # "push RegA"
                          }
                          frame 1 {
                            # "push RegB"
                          }
                          frame 2 {
                            # "push RegC"
                          }
                          frame 4 {
                            n199 = local read "AI1"() -> (w556:i16)
                          }
                        }
                        n200 = Number To Boolean Array(number=w540) -> (Boolean array=w544:bool[])
                        n201 = Index Array(array=w544, index=w539) -> (element=w543:bool)
                        n202 = Not(x=w543) -> (.not. x?=w542:bool)
                        n203 = Replace Array Subset(array=w544, new element=w542, index=w539) -> (w545:bool[])
                        n204 = Increment(x=w537) -> (x+1=w536:i16)
                        n205 = Boolean Array To Number(Boolean array=w545) -> (number=w541:u8)
                        n206 = xnode ("FIFO Write")("Element"=w547, "Timeout"=0) -> ()  [unwired: 1 in, 2 out]
                      }
                      frame 8 {
                        # "Stop and reset program"
                        n207 = Number To Boolean Array(number=w562) -> (Boolean array=w565:bool[])
                        n208 = Replace Array Subset(array=w565, new element=TRUE ("new element/subarray"), index=7) -> (w564:bool[])
                        n209 = Boolean Array To Number(Boolean array=w564) -> (number=w563:u8)
                      }
                      frame 9 {
                        # "Cold Lab Specific instructions"
                        n210 = case shown="1" w570 {
                          tunnel: w589 -> [w602 w607]
                          tunnel: w588 -> [w601 w606]
                          tunnel: w587 -> [w598 w608]
                          tunnel: [w598 w608] -> w586
                          tunnel: w585 -> [w597 w609]
                          tunnel: [w597 w609] -> w584
                          tunnel: w583 -> [w596 w610]
                          tunnel: [w596 w610] -> w582
                          tunnel: w581 -> [w595 w611]
                          tunnel: [w595 w611] -> w580
                          tunnel: w579 -> [w594 w612]
                          tunnel: [w594 w612] -> w578
                          tunnel: w577 -> [w593 w613]
                          tunnel: [w593 w613] -> w576
                          tunnel: [w592 w614] -> w575
                          tunnel: w574 -> [w592 w614]
                          tunnel: w573 -> [w591 w605]
                          tunnel: [w591 w605] -> w572
                          tunnel: w571 -> [_ w604]
                          tunnel: w570 -> [w590 _]
                          frame 0, Default {
                            # "Run Square wave generator"
                            n211 = Greater?(x=w590, y=u8 0) -> (0:w599:bool)
                            n212 = Join Numbers(hi=w602, lo=w601) -> ((hi.lo)=w603:u32)
                            n213 = local write "square wave  on?"(w599) -> ()
                            n214 = local write "square wave period"(w603) -> ()
                          }
                          frame 1 {
                            # "start compression"
                            n215 = Set Occurrence(w604) -> ()
                            n216 = local write "step size"(w606) -> ()
                            n217 = local write "End Current"(w607) -> ()
                          }
                        }
                      }
                      frame 10 {
                        n218 = local write "trigger AI1"(TRUE) -> ()
                      }
                    }
                    "control flags" <- w206
                    n219 = Number To Boolean Array(number=w206) -> (Boolean array=w215:bool[])
                    n220 = Index Array(array=w215, index=7) -> (element=w213:bool)
                    n221 = Or(x=w213, y="halt processor") -> (x .or. y?=w212:bool)
                    "IP address" <- w192
                    "ReA" <- w201
                    "RegB" <- w208
                    "RegC" <- w200
                    "FIFO size" <- w180
                    "RegD" <- w179
                  }
                  n222 = node-c288(w171) -> ()
                }
                frame True {
                }
              }
            }
          }
          frame #1 {
            n223 = local write "Run program"(FALSE ("Run program")) -> ()
          }
        }
      }
    }
  }
  n224 = while {
    tunnel: w1 -> [w633]
    stop <- FALSE stop-if-true
    n225 = flat-sequence {
      tunnel: w633 -> [w634]
      frame #0 {
        n226 = Wait on Occurrence(2:w634) -> ()  [unwired: 2 in, 1 out]
      }
      frame #1 {
        n227 = local read "AO0_pigeon"() -> (w635:i16)
        n228 = local write "AO0"(w635) -> ()
      }
    }
  }
  n229 = node-c288() -> (w8:T2)  [unwired: 1 in]
  n230 = while {
    shift-right: [w636] -> _
    shift-left: i16 0 -> [w637]
    stop <- FALSE stop-if-true
    n231 = case shown="False" "analog ramp on" {
      tunnel: [w640 w644] -> w636
      tunnel: w637 -> [w640 w641]
      frame False {
      }
      frame True {
        n232 = local read "analog ramp period"() -> (w643:i16)
        n233 = Less?(x=w641, y=w643) -> (x < y?=w642:bool)
        n234 = Increment(x=w641) -> (x+1=w645:i16)
        n235 = Not(x=w642) -> (.not. x?=w647:bool)
        n236 = Select(t=i16 0, s=w647, f=w645) -> (s? t:f=w644:i16)
        n237 = xnode "FPGA I/O Node"("Connector0/AO7"=w641) -> ()  [unwired: 1 in, 1 out]
        "Numeric" <- w641
      }
    }
  }
  n238 = while {
    stop <- FALSE stop-if-true
    n239 = xnode "FPGA I/O Node"() -> ("Connector0/AI0"=→"Connector0/AI0")  [unwired: 1 in, 1 out]
  }
  n240 = timed-loop {
    shift-right: [w651] -> _
    shift-left: u64 0 -> [w654]
    shift-right: [w653] -> _
    shift-left: TRUE -> [w652]
    timing: w8 -> [_]
    timing-out: [_] -> w7
    tunnel: [w653] -> _
    stop <- _ stop-if-true
    n241 = case shown="False" "square wave  on?" {
      tunnel: w654 -> [w656 w660]
      tunnel: [w655 w664] -> w653
      tunnel: w652 -> [w655 w663]
      tunnel: [w656 w661] -> w651
      frame False {
      }
      frame True {
        n242 = local read "square wave period"() -> (w659:i32)
        n243 = xnode "FPGA I/O Node"("Connector1/DIO6"=w663) -> ()  [unwired: 1 in, 1 out]
        n244 = Less?(x=w660, y=w659) -> (x < y?=w657:bool)
        n245 = Not(x=w657) -> (.not. x?=w658:bool)
        n246 = Increment(x=w660) -> (x+1=w666:u64)
        n247 = Not(x=w663) -> (.not. x?=w665:bool)
        n248 = Select(t=i16 0, s=w658, f=w666) -> (s? t:f=w661:u64)
        n249 = Greater Or Equal?(x=w661, y=w659) -> (x >= y?=w662:bool)
        n250 = Select(t=w665, s=w662, f=w663) -> (s? t:f=w664:bool)
      }
    }
  }
  n251 = node-c288(w7) -> ()
